vi "GOTO Z.vi"(5 "VMAX":dbl=600.0 format="%#_13g", 6 "reset":bool, 7 "ACC":dbl=800.0 format="%#_13g", 8 "error in (no error)":errorcluster, 11 "Z":dbl format="%#_13g") -> (0 "error out":errorcluster)   [LabVIEW 2018]
uses:
  <vilib>/Platform/TimedLoop/XDataNode/timing_clust.ctl
  <vilib>/Platform/TimedLoop/XDataNode/nitl_modes.ctl
  <vilib>/Platform/TimedLoop/XDataNode/wakeup.ctl
  <vilib>/platform/TimedLoop/XDataNode/XDataNode.xnode
  <vilib>/Platform/TimedLoop/XDataNode/XDNodeRunTimeDep.lvlib
  <vilib>/ptbypt/NI_PtbyPt.lvlib
panel:
  out "i":i32
  out "T3":dbl
  out "T1":dbl
  out "DC estimate (V)":dbl format="%0.2f"
  out "Waveform Chart":dbl(graph)
  out "theta":dbl
  out "x+y":dbl[](array[numeric])
  out "x*y":dbl
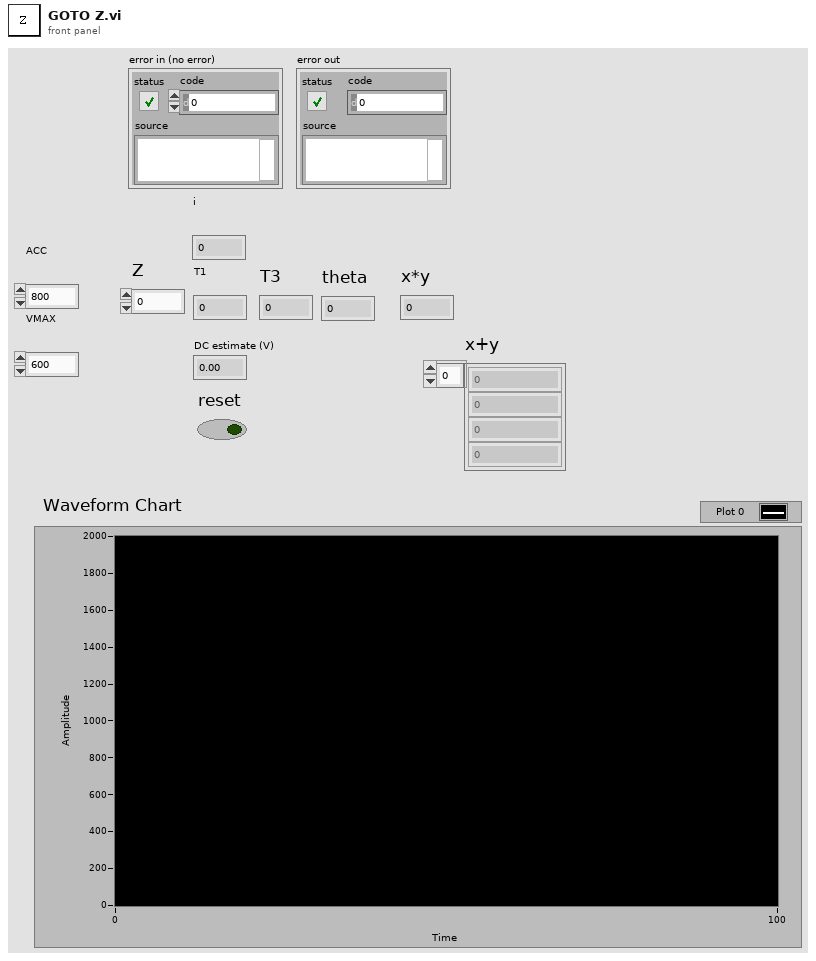
[diagram p1: front panel]
types:
  T1 = typedef "XDNodeRunTimeDep.lvlib/timing_clust.ctl" = cluster{"Expected End [f-1]":u64, "Actual End [f-1]":u64, "Finished Late? [f-1]":bool, "Expected End [i-1]":u64, "Actual End [i-1]":u64, "Finished Late? [i-1]":bool, "Expected Start [i]":u64, "Actual Start [i]":u64, "Expected Start [f]":u64, "Actual Start [f]":u64, "Source Name":string, "Structure Name":string, "Period":i64, "Deadline":i64, "Offset":i64, "Start":i64, "Priority":i32, "Timeout":i32, "Mode":T2, "Wakeup Reason":T3, "Error":errorcluster, "Source Type":string, "Secondary Source Type":string, "Global End Time":u64, "Global Start Time":u64, "Frame Duration":u64, "Iteration Duration":u64, "Assigned CPU":i32, "I/O Scan Engine Mode":u32}
  T2 = typedef "XDNodeRunTimeDep.lvlib/nitl_modes.ctl" = enum32{"No Change", "Process missed periods, maintain original phase", "Discard missed periods, maintain original phase", "Process missed periods, ignore original phase", "Discard missed periods, ignore original phase"}
  T3 = typedef "XDNodeRunTimeDep.lvlib/wakeup.ctl" = enum32{"Normal", "Aborted", "Asynchronous wakeup", "Timing source error", "Timed loop error", "Timeout"}
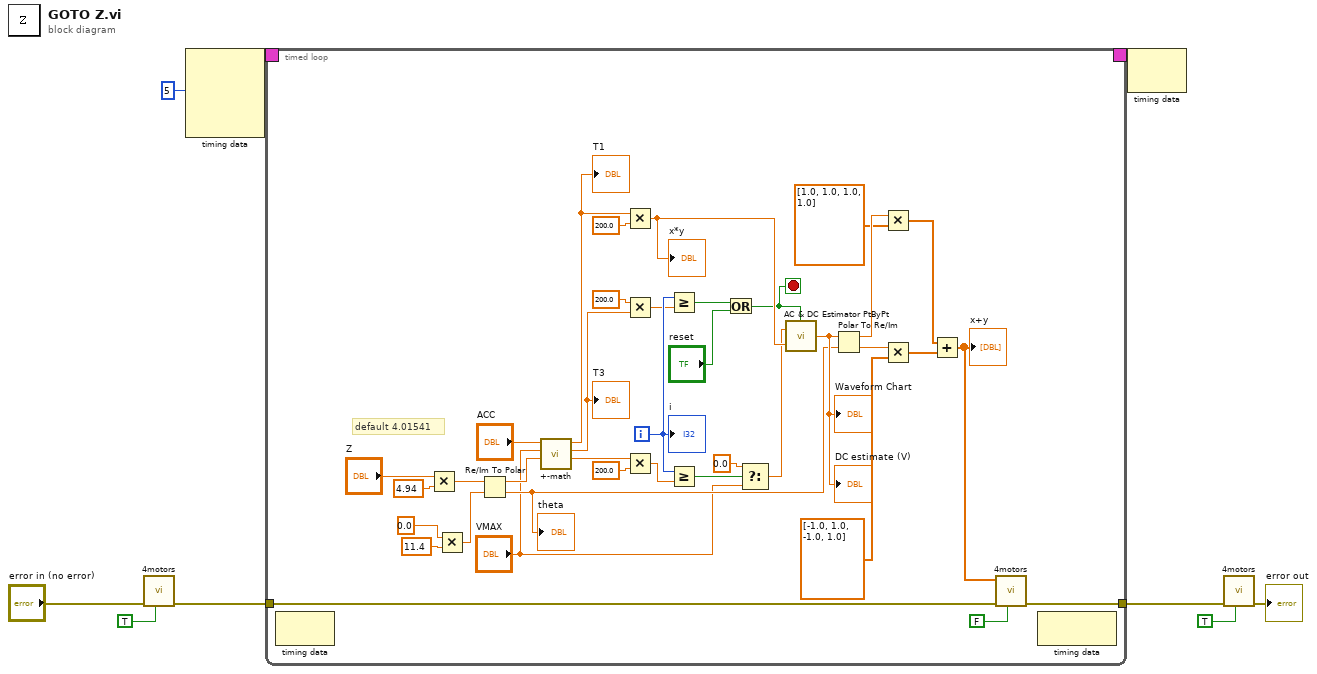
[diagram p0: block diagram]
diagram:
  n1 = call "4motors.vi"("Reset"=TRUE, "error in (no error)"="error in (no error)") -> ("error out"=w5:errorcluster)  [unwired: 8 in, 1 out]
  n2 = node-c288(i64 5 ("Period")) -> (w9:T1)  [unwired: 3 in]
  n3 = timed-loop {
    timing: w9 -> [_]
    timing-out: [_] -> w8
    tunnel: [w15] -> w6
    tunnel: w5 -> [w11]
    i -> [w21]
    stop <- w16 stop-if-true
    # "default 4.01541"
    n4 = node-c288() -> ()  [unwired: 1 in, 1 out]
    n5 = Multiply(x="Z", y=4.94) -> (x*y=w26:dbl)
    n6 = Multiply(x=0.0 ("Y"), y=11.4) -> (x*y=w23:dbl)
    n7 = Re/Im To Polar(2:w23, 3:w26) -> (0:w35:dbl, 1:w37:dbl)
    "theta" <- w35
    n8 = call "+-math.vi"("S"=w37, "VMAX"="VMAX", "ACC"="ACC") -> ("T2"=w42:dbl, "T3"=w12:dbl, "T1"=w45:dbl)  [unwired: 6 in]
    "T1" <- w45
    "T3" <- w12
    n9 = Multiply(x=w45, y=200.0) -> (x*y=w43:dbl)
    "x*y" <- w43
    n10 = Multiply(x=200.0, y=w12) -> (x*y=w20:dbl)
    n11 = Multiply(x=w42, y=200.0) -> (x*y=w40:dbl)
    n12 = Greater Or Equal?(x=w21, y=w20) -> (x >= y?=w19:bool)
    n13 = Greater Or Equal?(x=w21, y=w40) -> (x >= y?=w17:bool)
    n14 = Or(x=w19, y="reset") -> (x .or. y?=w16:bool)
    n15 = Select(t=0.0, s=w17, f="VMAX") -> (s? t:f=w38:dbl)
    n16 = call <vilib>:"AC & DC Estimator PtByPt.vi"("signal"=w38, "sample length"=w43, "initialize"=w16) -> ("DC estimate (V)"=w36:dbl)  [unwired: 2 out]
    "DC estimate (V)" <- w36
    "Waveform Chart" <- w36
    n17 = Polar To Re/Im(2:w35, 3:w36) -> (0:w32:dbl, 1:w34:dbl)
    n18 = Multiply(x=w34, y=dbl[] [1.0, 1.0, 1.0, 1.0]) -> (x*y=w30:dbl[])
    n19 = Multiply(x=w32, y=dbl[] [-1.0, 1.0, -1.0, 1.0]) -> (x*y=w29:dbl[])
    n20 = Add(x=w30, y=w29) -> (x+y=w13:dbl[])
    "x+y" <- w13
    n21 = call "4motors.vi"("Reset"=FALSE, "error in (no error)"=w11, "Power"=w13) -> ("error out"=w15:errorcluster)  [unwired: 7 in, 1 out]
    n22 = node-c288() -> ()  [unwired: 1 in, 1 out]
    "i" <- w21
  }
  n23 = node-c288(w8) -> ()  [unwired: 1 out]
  n24 = call "4motors.vi"("Reset"=TRUE, "error in (no error)"=w6) -> ("error out"=→"error out":errorcluster)  [unwired: 8 in, 1 out]
